vi "MotionProfileControlsInit.vi"() -> (0 "MotionPlanningNotifiers":T1)   [LabVIEW 2018]
uses:
  TypeDefs/RobotComponents/MotionPlanningNotifiers.ctl
  Implements/Arm/TypeDefs/ArmPlanRequest.ctl
  Implements/Arm/TypeDefs/ArmTargetPosition.ctl
  Implements/Arm/TypeDefs/ArmPlanResponse.ctl
  General/MotionProfiling/TypeDefs/TrajectoryPoint.ctl
  <vilib>/Rock Robotics/WPI/ThirdParty/Phoenix-LabVIEW/Motor Controller/Controls/CTRE_Phoenix_MotorControl_TrajectoryPointTimeDur.ctl
  General/MotionProfiling/TypeDefs/ArmMotionProfileControl.ctl
  MotionProfileControlData.vi
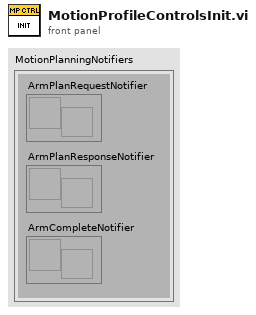
[diagram p1: front panel]
types:
  T1 = typedef "MotionPlanningNotifiers.ctl" = cluster{"ArmPlanRequestNotifier":refnum<notifier>, "ArmPlanResponseNotifier":refnum<notifier>, "ArmCompleteNotifier":refnum<notifier>}
  T2 = typedef "ArmMotionProfileControl.ctl" = cluster{"ControlMutex":T3, "Trajectory Points":T4[], "CurrentIndex":u32}
  T3 = typedef "Semaphore RefNum" = refnum<k1>
  T4 = typedef "TrajectoryPoint.ctl" = cluster{"Position ":dbl, "Velocity ":dbl, "Time (ms)":T5, "Last Point":bool}
  T5 = typedef "CTRE_Phoenix_MotorControl_TrajectoryPointTimeDur.ctl" = i32
  T6 = typedef "ArmPlanResponse.ctl" = cluster{"ShoulderTrajectory":T4[], "ExtendTrajectory":T4[], "PlanTime (ms)":u32, "Execute":bool, "WristTrajectory":T4[]}
  T7 = typedef "ArmPlanRequest.ctl" = cluster{"Destination":T8, "Preview":bool, "Start":T8, "Fixed Start":bool}
  T8 = typedef "ArmTargetPosition.ctl" = enum16{"Forward Cargo Hold", "Forward Cargo Low", "Forward Cargo Middle", "Forward Cargo High", "Forward Hatch Hold", "Forward Hatch Low", "Forward Hatch Middle", "Forward Hatch High", "Reverse Cargo Hold", "Reserve Cargo Low", "Reverse Cargo Middle", "Reverse Cargo High", "Reverse Hatch Hold", "Reverse Hatch Low", "Reverse Hatch Middle", "Reverse Hatch High"}
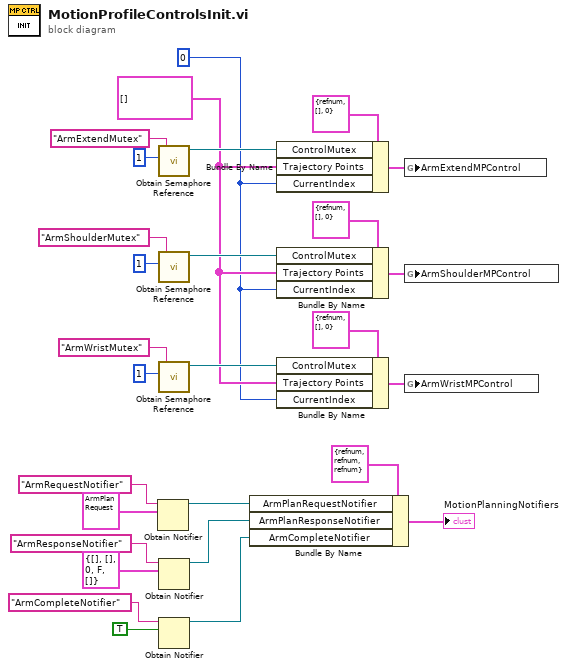
[diagram p0: block diagram]
diagram:
  w1 = u32 0 ("ArmExtendMPControl.CurrentIndex")
  w2 = T4[] [] ("ArmExtendMPControl.Trajectory Points")
  n1 = Obtain Notifier(name (unnamed)="ArmRequestNotifier", notification data type=T7 {"Destination"=enum."Forward Cargo Hold", "Preview"=FALSE, "Start"=enum."Forward Cargo Hold", "Fixed Start"=FALSE} ("ArmPlanRequest")) -> (notifier out=w16:refnum<notifier>)  [unwired: 2 in, 2 out]
  n2 = call <vilib>:"Obtain Semaphore Reference.vi"("size (1)"=1, "name (unnamed)"="ArmExtendMutex") -> ("semaphore"=w28:T3)  [unwired: 3 in, 2 out]
  n3 = call <vilib>:"Obtain Semaphore Reference.vi"("size (1)"=1, "name (unnamed)"="ArmShoulderMutex") -> ("semaphore"=w21:T3)  [unwired: 3 in, 2 out]
  n4 = call <vilib>:"Obtain Semaphore Reference.vi"("size (1)"=1, "name (unnamed)"="ArmWristMutex") -> ("semaphore"=w6:T3)  [unwired: 3 in, 2 out]
  n5 = Obtain Notifier(name (unnamed)="ArmResponseNotifier", notification data type=T6 {"ShoulderTrajectory"=[], "ExtendTrajectory"=[], "PlanTime (ms)"=0, "Execute"=FALSE, "WristTrajectory"=[]} ("ArmPlanResponse")) -> (notifier out=w15:refnum<notifier>)  [unwired: 2 in, 2 out]
  n6 = Obtain Notifier(name (unnamed)="ArmCompleteNotifier", notification data type=TRUE) -> (notifier out=w8:refnum<notifier>)  [unwired: 2 in, 2 out]
  n7 = Bundle By Name(cluster=T1 {"ArmPlanRequestNotifier"=refnum, "ArmPlanResponseNotifier"=refnum, "ArmCompleteNotifier"=refnum} ("MotionPlanningNotifiers"), "ArmPlanRequestNotifier"=w16, "ArmPlanResponseNotifier"=w15, "ArmCompleteNotifier"=w8) -> (→"MotionPlanningNotifiers":T1)
  n8 = Bundle By Name(cluster=T2 {"ControlMutex"=refnum, "Trajectory Points"=[], "CurrentIndex"=0} ("MotionProfileControl"), "ControlMutex"=w28, "Trajectory Points"=w2, "CurrentIndex"=w1) -> (w25:T2)
  n9 = Bundle By Name(cluster=T2 {"ControlMutex"=refnum, "Trajectory Points"=[], "CurrentIndex"=0} ("MotionProfileControl"), "ControlMutex"=w21, "Trajectory Points"=w2, "CurrentIndex"=w1) -> (w22:T2)
  n10 = Bundle By Name(cluster=T2 {"ControlMutex"=refnum, "Trajectory Points"=[], "CurrentIndex"=0} ("MotionProfileControl"), "ControlMutex"=w6, "Trajectory Points"=w2, "CurrentIndex"=w1) -> (w5:T2)
  n11 = global write "MotionProfileControlData.vi" "ArmExtendMPControl"(w25) -> ()
  n12 = global write "MotionProfileControlData.vi" "ArmShoulderMPControl"(w22) -> ()
  n13 = global write "MotionProfileControlData.vi" "ArmWristMPControl"(w5) -> ()
